vi "Receive (I2S).vi"(6 "ready for output":bool, 7 "configuration":T1={"bits per channel"=2, "data sample edge"=enum."falling", "inverted sync"=FALSE}, 9 "receive":bool, 11 "signals in":cluster{"clock":bool, "sync":bool, "sdata":bool}) -> (1 "output valid":bool, 3 "sample":u32)   [LabVIEW 2013, in "I2S-TDM.lvlib"]
uses:
  I2S-TDM.lvlib
  Controls/i2s receiver configuration.ctl
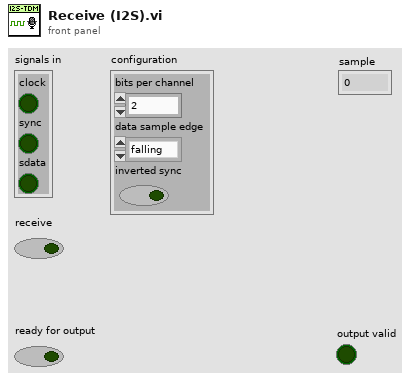
[diagram p1: front panel]
types:
  T1 = typedef "I2S-TDM.lvlib/i2s receiver configuration.ctl" = cluster{"bits per channel":u8, "data sample edge":enum16{"rising", "falling"}, "inverted sync":bool}
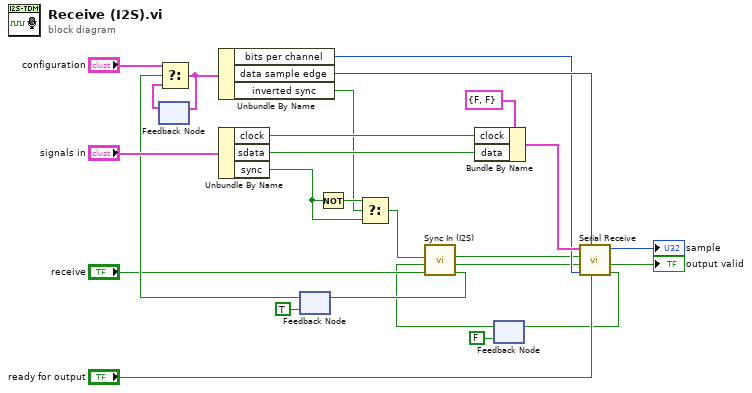
[diagram p0: block diagram]
diagram:
  n1 = feedback #1() -> (w13:T1)  [unwired: 1 in]
  n2 = Unbundle By Name("signals in") -> ("clock"=w24:bool, "sdata"=w23:bool, "sync"=w19:bool)
  n3 = feedback #2(TRUE ("latch config")) -> (w12:bool)
  n4 = Select(t="configuration", s=w12, f=w13) -> (s? t:f=w14:T1)
  n5 = feedback-in #1(w14) -> ()
  n6 = Unbundle By Name(w14) -> ("bits per channel"=w16:u8, "data sample edge"=w21:enum16{"rising", "falling"}, "inverted sync"=w17:bool)
  n7 = Not(x=w19) -> (.not. x?=w18:bool)
  n8 = Select(t=w18, s=w17, f=w19) -> (s? t:f=w1:bool)
  n9 = Bundle By Name(cluster=cluster{"clock":bool, "data":bool} {"clock"=FALSE, "data"=FALSE} ("signals in"), "clock"=w24, "data"=w23) -> (w22:cluster{"clock":bool, "data":bool})
  n10 = feedback #3(FALSE ("latch config")) -> (w2:bool)
  n11 = call "Sync In (I2S).vi"("receive"="receive", "prev transfer done"=w2, "sync in"=w1) -> ("latch config"=w6:bool, "force output"=w5:bool, "start read"=w4:bool)  [unwired: 6 in]
  n12 = feedback-in #2(w6) -> ()
  n13 = call "Serial Receive.vi"("ready for output"="ready for output", "data sampling edge"=w21, "transfer length"=w16, "force output (F)"=w5, "start transfer"=w4, "signals in"=w22) -> ("transfer done"=w8:bool, "output valid"=→"output valid":bool, "sample out"=→"sample":u32)  [unwired: 3 in]
  n14 = feedback-in #3(w8) -> ()
